vi "TDMS Log Loop.vi"(8 "error in (no error)":errorcluster, 11 "Message Queues":T1) -> (0 "error out":errorcluster)   [LabVIEW 2021, in "TDMS Log.lvlib"]
uses:
  TDMS Log.lvlib
  Main/Main Queue Cluster.ctl
  support/Message Queue/Message Cluster.ctl
  TDMS Log State Cluster.ctl
  support/Message Queue/Enqueue Message (Single).vi
  support/Message Queue/Message Queue.lvlib
  Waveform Loop/Waveform Loop.lvlib
  support/Command Log VIs/Command Logging.lvlib
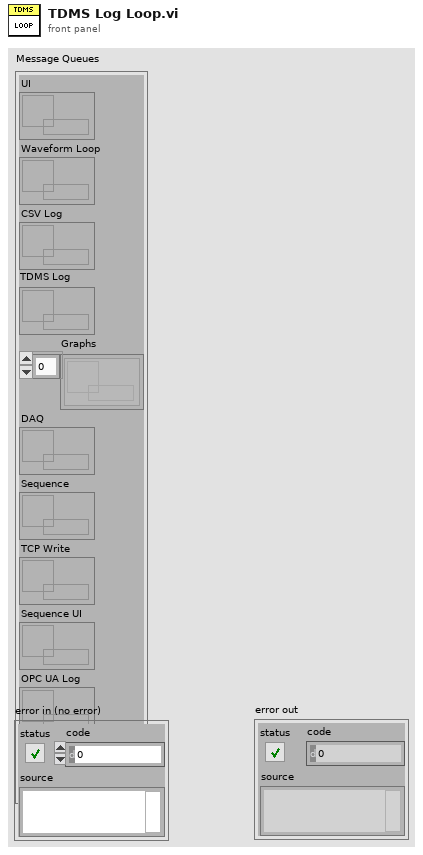
[diagram p1: front panel]
types:
  T1 = typedef "Main Queue Cluster.ctl" = cluster{"UI":refnum<queue>, "Waveform Loop":refnum<queue>, "CSV Log":refnum<queue>, "TDMS Log":refnum<queue>, "Graphs":refnum<queue>[], "DAQ":refnum<queue>, "Sequence":refnum<queue>, "TCP Write":refnum<queue>, "Sequence UI":refnum<queue>, "OPC UA Log":refnum<queue>, "TCP Read":refnum<queue>}
  T2 = typedef "TDMS Log.lvlib/TDMS Log State Cluster.ctl" = cluster{"TDMS log path":path, "tdms file":refnum<k34>}
  T3 = enum16{"open", "open or create", "create or replace", "create", "open (read-only)"}
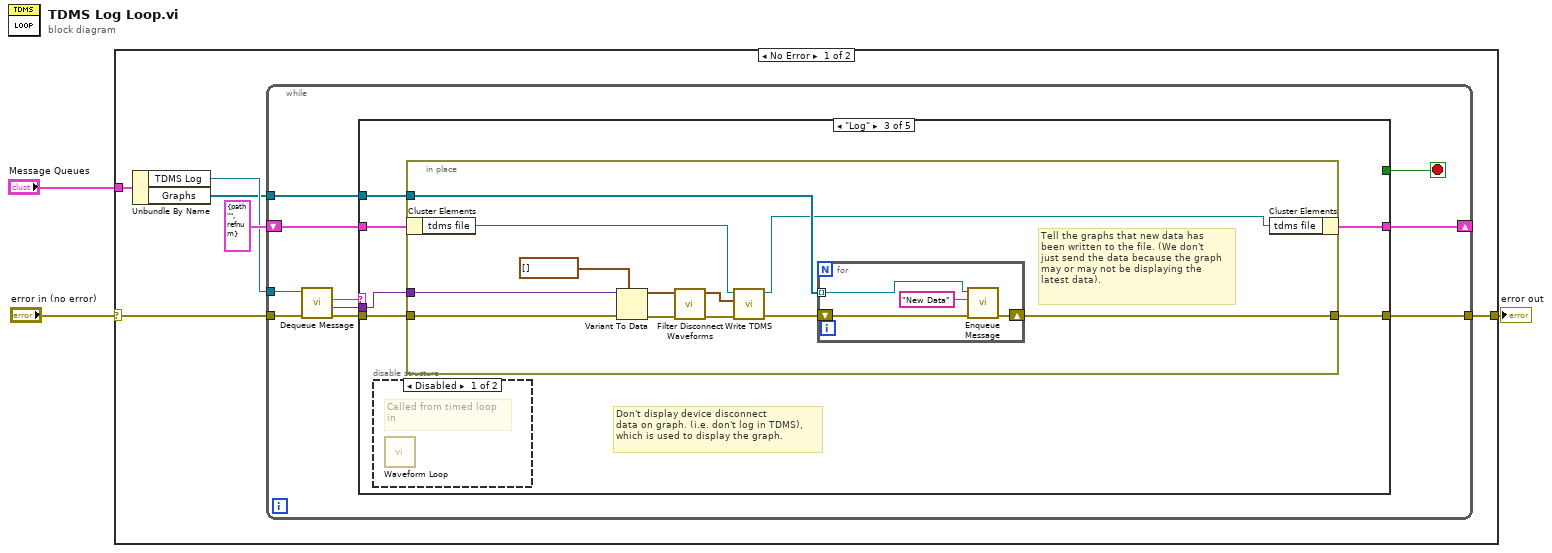
[diagram p0: block diagram]
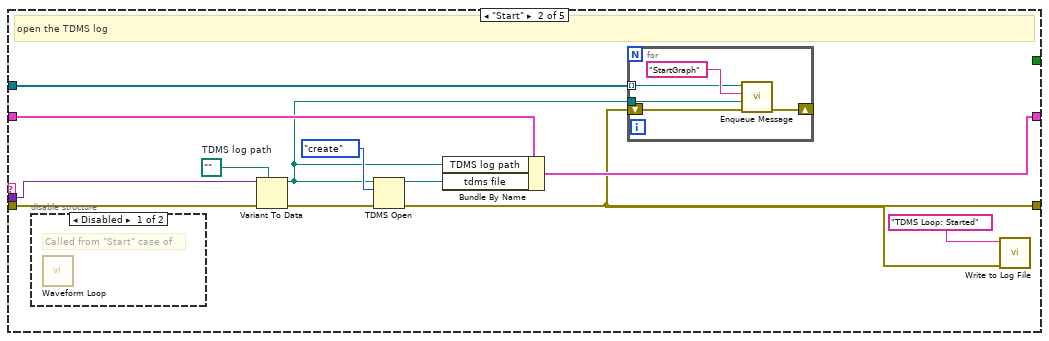
[diagram p3: hidden frame]
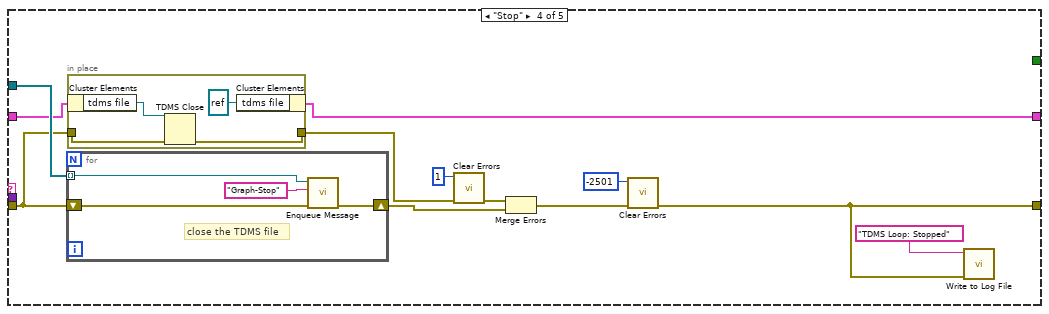
[diagram p6: hidden frame]
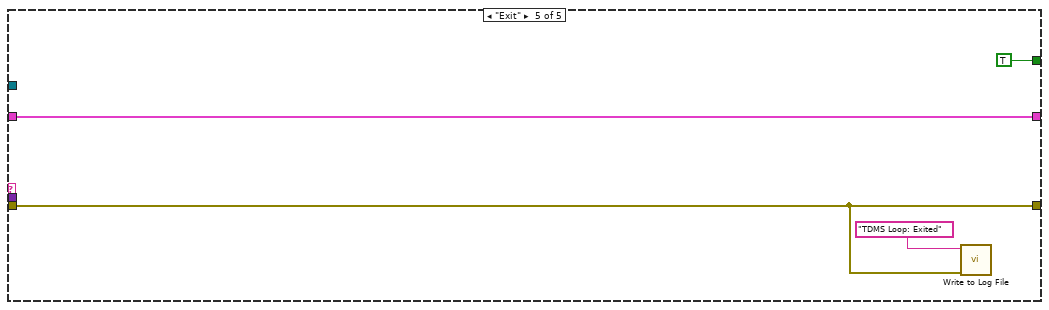
[diagram p7: hidden frame]
diagram:
  n1 = case shown="No Error" "error in (no error)" {
    selector: "error in (no error)" -> [w4 w85]
    tunnel: "Message Queues" -> [w8 _]
    tunnel: [w5 w85] -> w2
    frame No Error {
      n2 = Unbundle By Name(w8) -> ("TDMS Log"=w7:refnum<queue>, "Graphs"=w6:refnum<queue>[])
      n3 = while {
        shift-right: [w16] -> _
        shift-left: T2 {"TDMS log path"=path "", "tdms file"=refnum} ("Waveform Loop State") -> [w18]
        tunnel: w7 -> [w13]
        tunnel: w6 -> [w12]
        tunnel: w4 -> [w11]
        tunnel: [w10] -> w5
        stop <- w14 stop-if-true
        n4 = call "Dequeue Message.vi"("error in (no error)"=w11, "Message Queue"=w13) -> ("error out"=w15:errorcluster, "Message Data"=w17:variant, "Message"=w19:string)  [unwired: 6 in, 1 out]
        n5 = case shown="\"Log\"" w19 {
          tunnel: w18 -> [w21 w33 w40 w62 w84]
          tunnel: w17 -> [_ w32 w43 _ _]
          tunnel: [w21 w31 w39 w61 w84] -> w16
          tunnel: w15 -> [w20 w26 w44 w71 w81]
          tunnel: [_ _ _ _ TRUE] -> w14
          tunnel: [w20 w22 w41 w67 w81] -> w10
          tunnel: w12 -> [_ w25 w42 w72 _]
          frame Default {
            # "This case should not be called"
          }
          frame "Start" {
            w30 = path ""  # TDMS log path
            # "open the TDMS log"
            n6 = disable-structure shown="Disabled" {
              frame Disabled {
                # "Called from \"Start\" case of"
                n7 = call "Waveform Loop.vi"() -> ()  [unwired: 11 in, 1 out]
              }
              frame Enabled {
              }
            }
            n8 = Variant To Data(error in=w26, type=w30, Variant=w32) -> (data=w24:path, error out=w27:errorcluster)
            n9 = TDMS Open(8:w27, 10:T3."create" ("operation (0:open)"), 11:w24) -> (0:w22:errorcluster, 3:w29:refnum<k34>)  [unwired: 4 in]
            n10 = Bundle By Name(cluster=w33, "TDMS log path"=w24, "tdms file"=w29) -> (w31:T2)
            n11 = for {
              tunnel: w25 -> [w37] mode=indexing
              tunnel: w24 -> [w36]
              shift-right: [w34] -> _
              shift-left: w22 -> [w35]
              n12 = call-poly "Enqueue Message.vi"("error in (no error)"=w35, "Message Data"=w36, "Message"="StartGraph", "Message Queue"=w37) -> ("error out"=w34:errorcluster)  [unwired: 6 in, 1 out]
            }
            n13 = call "Write to Log File.vi"("error in"=w22, "text"="TDMS Loop: Started") -> ()  [unwired: 9 in, 1 out]
          }
          frame "Log" {
            # "Don't display device disconnect\ndata on graph. (i.e. don't log in TDMS),\nwhich is used to display the graph."
            n14 = disable-structure shown="Disabled" {
              frame Disabled {
                # "Called from timed loop\nin"
                n15 = call "Waveform Loop.vi"() -> ()  [unwired: 11 in, 1 out]
              }
              frame Enabled {
              }
            }
            n16 = in-place {
              in-place-border: w44 -> [w56]
              in-place-border: w43 -> [w55]
              in-place-border: w42 -> [w53]
              in-place-border: [w47] -> w41
              # "Tell the graphs that new data has\nbeen written to the file. (We don't\njust send the data because the graph\nmay or may not be displaying the\nlatest data)."
              n17 = in-place-cluster #1(w40) -> ("tdms file"=w46:refnum<k34>)
              n18 = Variant To Data(error in=w56, type=waveform(dbl)[] [], Variant=w55) -> (data=w51:waveform(dbl)[], error out=w49:errorcluster)
              n19 = call "Filter Disconnect Waveforms.vi"("error in (no error)"=w49, "Waveform array in"=w51) -> ("error out"=w48:errorcluster, "Waveform array out"=w50:waveform(dbl)[])  [unwired: 8 in]
              n20 = call "Write TDMS.vi"("error in (no error)"=w48, "Array"=w50, "Refnum in"=w46) -> ("error out"=w52:errorcluster, "Refnum out"=w45:refnum<k34>)  [unwired: 7 in]
              n21 = for {
                tunnel: w53 -> [w59] mode=indexing
                shift-right: [w57] -> w47
                shift-left: w52 -> [w58]
                n22 = call-poly "Enqueue Message.vi"("error in (no error)"=w58, "Message"="New Data", "Message Queue"=w59) -> ("error out"=w57:errorcluster)  [unwired: 7 in, 1 out]
              }
              n23 = in-place-cluster #1("tdms file"=w45) -> (w39:T2)
            }
          }
          frame "Stop" {
            n24 = for {
              tunnel: w72 -> [w79] mode=indexing
              shift-right: [w77] -> w70
              shift-left: w71 -> [w78]
              # "close the TDMS file"
              n25 = call-poly "Enqueue Message.vi"("error in (no error)"=w78, "Message"="Graph-Stop", "Message Queue"=w79) -> ("error out"=w77:errorcluster)  [unwired: 7 in, 1 out]
            }
            n26 = in-place {
              in-place-border: w71 -> [w76]
              in-place-border: [w75] -> w64
              n27 = in-place-cluster #2(w62) -> ("tdms file"=w74:refnum<k34>)
              n28 = TDMS Close(8:w76, 11:w74) -> (0:w75:errorcluster)  [unwired: 1 out]
              n29 = in-place-cluster #2("tdms file"=refnum<k34> refnum) -> (w61:T2)
            }
            n30 = call <vilib>:"Clear Errors.vi"("error in (no error)"=w64, "specific error code to clear (0: all)"=1) -> ("error out"=w63:errorcluster)  [unwired: 4 in, 1 out]
            n31 = Merge Errors(w63, w70) -> (w68:errorcluster)
            n32 = call <vilib>:"Clear Errors.vi"("error in (no error)"=w68, "specific error code to clear (0: all)"=-2501) -> ("error out"=w67:errorcluster)  [unwired: 4 in, 1 out]
            n33 = call "Write to Log File.vi"("error in"=w67, "text"="TDMS Loop: Stopped") -> ()  [unwired: 9 in, 1 out]
          }
          frame "Exit" {
            n34 = call "Write to Log File.vi"("error in"=w81, "text"="TDMS Loop: Exited") -> ()  [unwired: 9 in, 1 out]
          }
        }
      }
    }
    frame Error {
    }
  }
  "error out" <- w2
